vi "BIT-BASH test toplevel.vi"() -> ()   [LabVIEW 2012]
uses:
  <vilib>/rvi/eio/common/nirviEmuTemplateMethod_errors.vi
  <vilib>/eio/EIONode/EIONode.xnode
  <vilib>/eio/EIOMethodNode/EIOMethodNode.xnode
panel:
  out "Data out":u8 format="%.0x"
  in  "Read Address":u8 format="%.0x"
  in  "Read?":bool
  in  "Write?":bool
  in  "Data In":u8 format="%.0x"
  in  "Write Address":u8 format="%.0x"
  in  "stop":bool
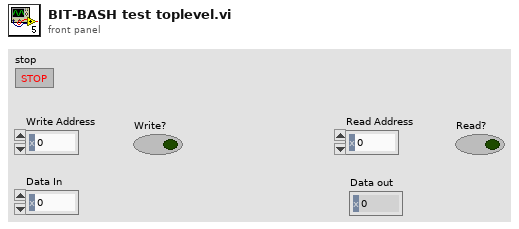
[diagram p1: front panel]
types:
  T1 = cluster{"SCK":refnum<k21>, "MISO":refnum<k21>, "MOSI":refnum<k21>, "CS":refnum<k21>}
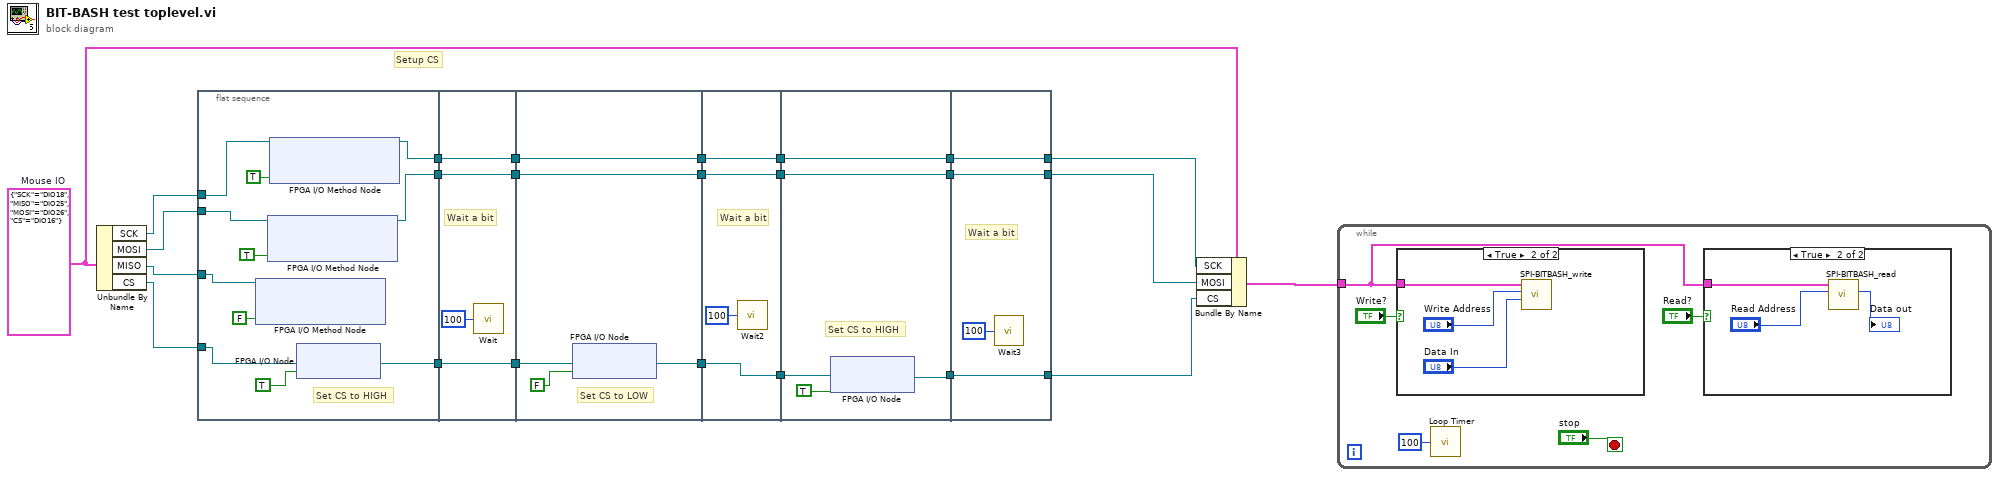
[diagram p0: block diagram]
diagram:
  w11 = T1 {"SCK"="DIO18", "MISO"="DIO25", "MOSI"="DIO26", "CS"="DIO16"}  # Mouse IO
  # "Setup CS"
  n1 = Unbundle By Name(w11) -> ("SCK"=w15:refnum<k21>, "MOSI"=w14:refnum<k21>, "MISO"=w13:refnum<k21>, "CS"=w12:refnum<k21>)
  n2 = flat-sequence {
    tunnel: w14 -> [w35]
    tunnel: w15 -> [w32]
    tunnel: w13 -> [w29]
    tunnel: w12 -> [w27]
    tunnel: [w33] -> w24
    tunnel: [w31] -> w23
    tunnel: [w25] -> w22
    tunnel: w24 -> [w39]
    tunnel: w23 -> [w38]
    tunnel: [w39] -> w21
    tunnel: [w38] -> w20
    tunnel: [w36] -> w19
    tunnel: w22 -> [w36]
    tunnel: w21 -> [w44]
    tunnel: w20 -> [w43]
    tunnel: w19 -> [w41]
    tunnel: [w44] -> w18
    tunnel: [w43] -> w17
    tunnel: [w40] -> w16
    tunnel: w18 -> [w48]
    tunnel: w17 -> [w47]
    tunnel: w16 -> [w45]
    tunnel: [w48] -> w6
    tunnel: [w47] -> w5
    tunnel: [w45] -> w4
    tunnel: w6 -> [w53]
    tunnel: w5 -> [w52]
    tunnel: w4 -> [w51]
    tunnel: [w53] -> w3
    tunnel: [w52] -> w2
    tunnel: [w50] -> w1
    tunnel: [w55] -> w8
    tunnel: [w56] -> w10
    tunnel: [w57] -> w9
    tunnel: w3 -> [w57]
    tunnel: w2 -> [w56]
    tunnel: w1 -> [w55]
    frame #0 {
      # "Set CS to HIGH"
      n3 = xnode "FPGA I/O Method Node"("FPGA I/O In"=w29, "Enable"=FALSE) -> ()  [unwired: 1 out]
      n4 = xnode "FPGA I/O Method Node"("FPGA I/O In"=w35, "Enable"=TRUE) -> ("FPGA I/O Out"=w33:refnum<k21>)
      n5 = xnode "FPGA I/O Method Node"("FPGA I/O In"=w32, "Enable"=TRUE) -> ("FPGA I/O Out"=w31:refnum<k21>)
      n6 = xnode "FPGA I/O Node"("I/O Item"=TRUE, "FPGA I/O In"=w27) -> ("FPGA I/O Out"=w25:refnum<k21>)
    }
    frame #1 {
      # "Wait a bit"
      n7 = call "Wait"("Count(uSec)"=u32 100) -> ()  [unwired: 1 out]
    }
    frame #2 {
      # "Set CS to LOW"
      n8 = xnode "FPGA I/O Node"("I/O Item"=FALSE, "FPGA I/O In"=w41) -> ("FPGA I/O Out"=w40:refnum<k21>)
    }
    frame #3 {
      # "Wait a bit"
      n9 = call "Wait2"("Count(uSec)"=u32 100) -> ()  [unwired: 1 out]
    }
    frame #4 {
      # "Set CS to HIGH"
      n10 = xnode "FPGA I/O Node"("I/O Item"=TRUE, "FPGA I/O In"=w51) -> ("FPGA I/O Out"=w50:refnum<k21>)
    }
    frame #5 {
      # "Wait a bit"
      n11 = call "Wait3"("Count(uSec)"=u32 100) -> ()  [unwired: 1 out]
    }
  }
  n12 = Bundle By Name(cluster=w11, "SCK"=w10, "MOSI"=w9, "CS"=w8) -> (w7:T1)
  n13 = while {
    tunnel: w7 -> [w58]
    stop <- "stop" stop-if-true
    n14 = case shown="True" "Write?" {
      tunnel: w58 -> [_ w68]
      frame False {
      }
      frame True {
        n15 = call "SPI-BITBASH_write.vi"("Data In"="Data In", "Write Address"="Write Address", "Mouse IO"=w68) -> ()  [unwired: 8 in, 1 out]
      }
    }
    n16 = call "Loop Timer"("Count(mSec)"=u32 100) -> ()  [unwired: 1 out]
    n17 = case shown="True" "Read?" {
      tunnel: w58 -> [_ w65]
      frame False {
      }
      frame True {
        n18 = call "SPI-BITBASH_read.vi"("Read Address"="Read Address", "Mouse IO"=w65) -> ("Data out"=→"Data out":u8)  [unwired: 8 in, 1 out]
      }
    }
  }
